vi "stitch interpolated images2.vi"(9 "DeltaE":dbl, 10 "Array of images to stitch":cluster{dbl[][]}[](array[cluster]), 11 "calib \"final\"":T1[](array[typedef])) -> (3 "stitched array image":sgl[][](array[numeric]))   [LabVIEW 2013]
uses:
  Controls/finalCalib--Cluster.ctl
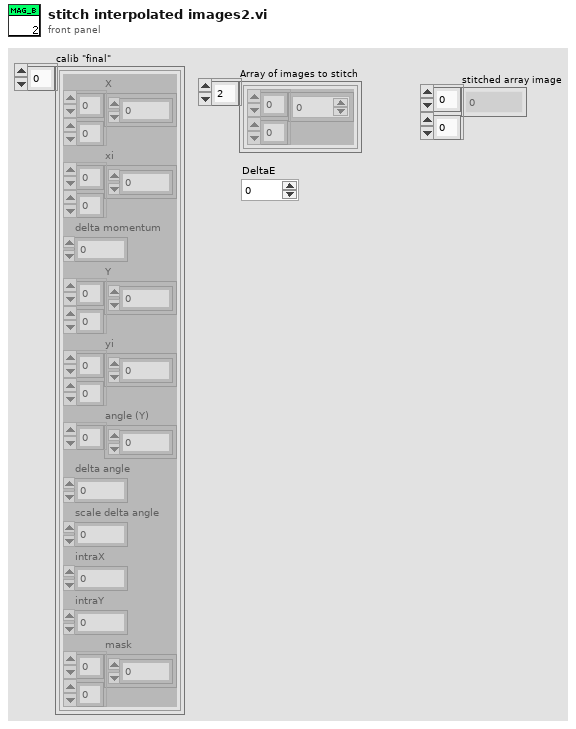
[diagram p1: front panel]
types:
  T1 = typedef "finalCalib--Cluster.ctl" = cluster{"X":dbl[][], "xi":dbl[][], "delta momentum":dbl, "Y":dbl[][], "yi":dbl[][], "angle (Y)":dbl[], "delta angle":dbl, "scale delta angle":dbl, "intraX":dbl, "intraY":dbl, "mask":dbl[][]}
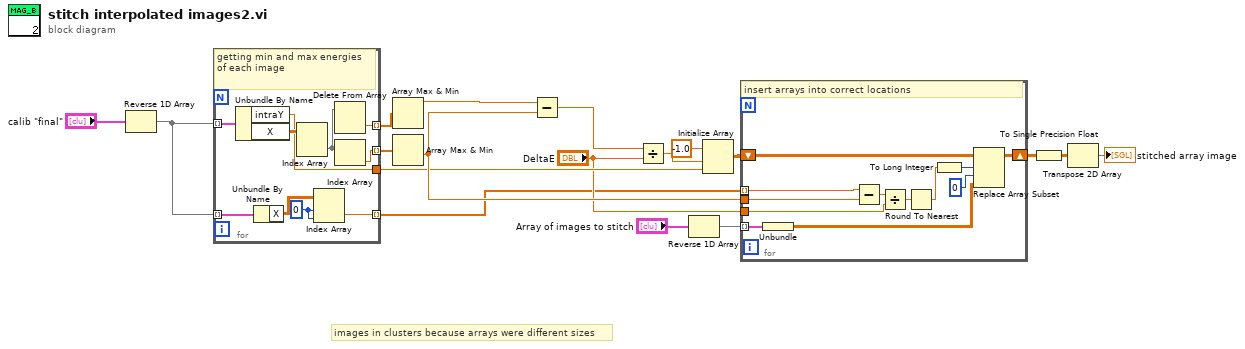
[diagram p0: block diagram]
diagram:
  # "images in clusters because arrays were different sizes"
  n1 = Reverse 1D Array(array="calib \"final\"") -> (reversed array=w2:T1[])
  n2 = for {
    tunnel: w2 -> [w28] mode=indexing
    tunnel: [w25] -> w7 mode=indexing
    tunnel: [w24] -> w6 mode=indexing
    tunnel: [w23] -> w10
    tunnel: w2 -> [w20] mode=indexing
    tunnel: [w19] -> w1 mode=indexing
    w22 = 0 ("disabled index (row)")
    # "getting min and max energies of each image"
    n3 = Unbundle By Name(w28) -> ("intraY"=w23:dbl, "X"=w27:dbl[][])
    n4 = Unbundle By Name(w20) -> ("X"=w21:dbl[][])
    n5 = Index Array(array=w27) -> (element=w26:dbl[])  [unwired: 2 in]
    n6 = Index Array(array=w21, index (row)=w22, index (col)=w22) -> (element=w19:dbl)
    n7 = Delete From Array(array=w26) -> (deleted portion=w25:dbl)  [unwired: 2 in, 1 out]
    n8 = Index Array(array=w26) -> (element=w24:dbl)  [unwired: 1 in]
  }
  n9 = Array Max & Min(array=w7) -> (max value=w8:dbl)  [unwired: 3 out]
  n10 = Array Max & Min(array=w6) -> (min value=w13:dbl)  [unwired: 3 out]
  n11 = Subtract(x=w8, y=w13) -> (x-y=w17:dbl)
  n12 = Divide(x=w17, y="DeltaE") -> (x/y=w18:dbl)
  n13 = Reverse 1D Array(array="Array of images to stitch") -> (reversed array=w12:cluster{dbl[][]}[])
  n14 = Initialize Array(-1.0, w18, w10) -> (w11:dbl[][])
  n15 = for {
    tunnel: "DeltaE" -> [w35]
    shift-right: [w34] -> w14
    shift-left: w11 -> [w40]
    tunnel: w12 -> [w39] mode=indexing
    tunnel: w13 -> [w37]
    tunnel: w1 -> [w29] mode=indexing
    # "insert arrays into correct locations"
    n16 = Unbundle(w39) -> (w38:dbl[][])
    n17 = Subtract(x=w29, y=w37) -> (x-y=w36:dbl)
    n18 = Divide(x=w36, y=w35) -> (x/y=w32:dbl)
    n19 = Round To Nearest(number=w32) -> (nearest integer value=w33:dbl)
    n20 = To Long Integer(number=w33) -> (32bit integer=w31:i32)
    n21 = Replace Array Subset(array=w40, new element=w38, index (row)=w31, index (col)=0 ("disabled index (row)")) -> (w34:dbl[][])
  }
  n22 = To Single Precision Float(number=w14) -> (single precision float=w15:sgl[][])
  n23 = Transpose 2D Array(2D array=w15) -> (transposed array=→"stitched array image":sgl[][])
